vi "Last_L1_FolderName.vi"(11 "folder names":string[](array[string])) -> (3 "File_Name":string[](array[string]))   [LabVIEW 2023]
panel:
  out "Times":i64[](array[numeric])
  out "Name-SN":string[](array[string])
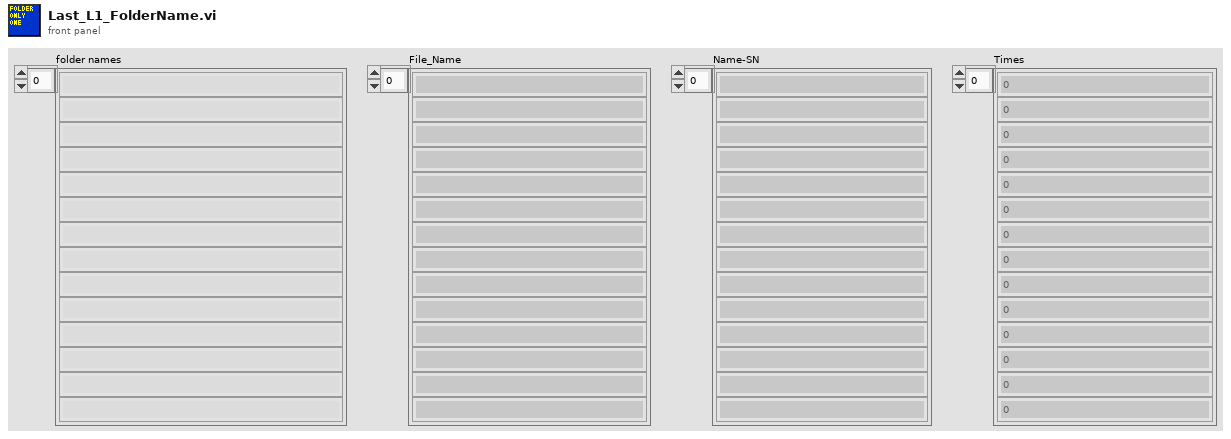
[diagram p1: front panel]
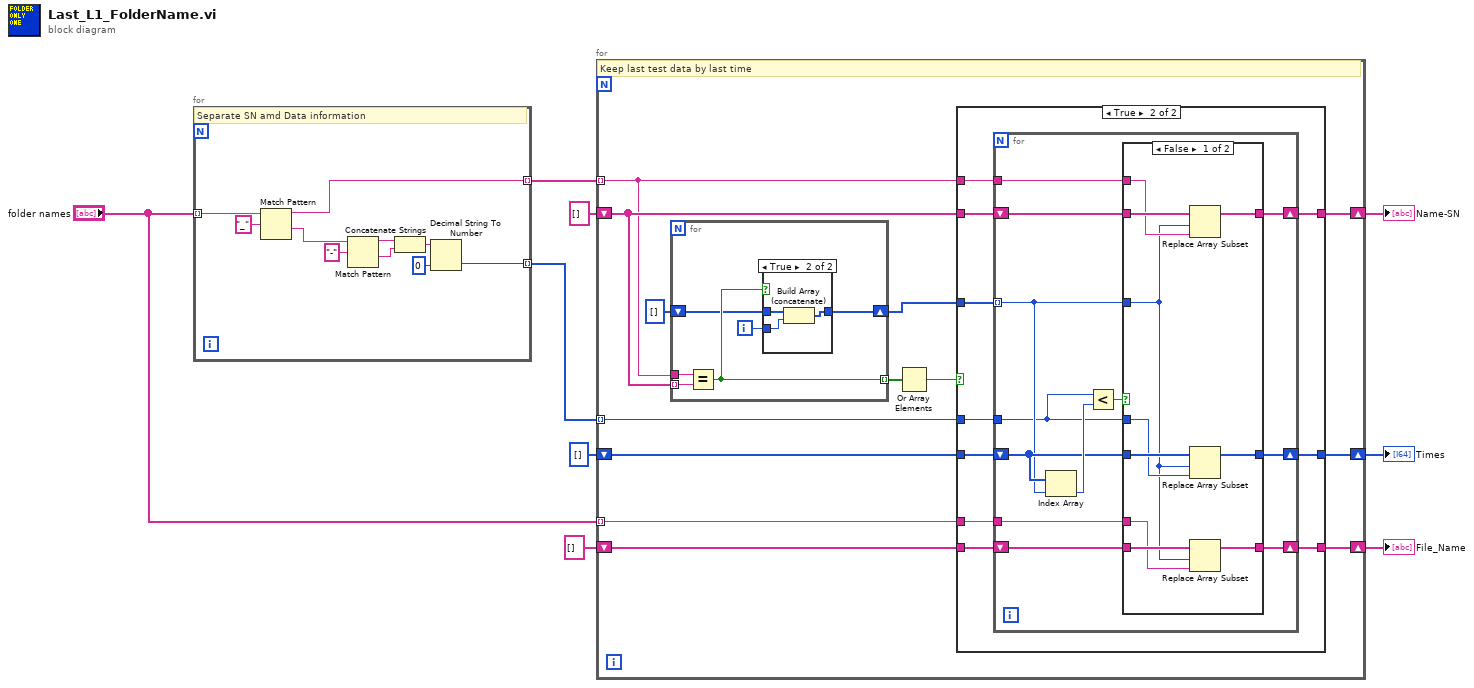
[diagram p0: block diagram]
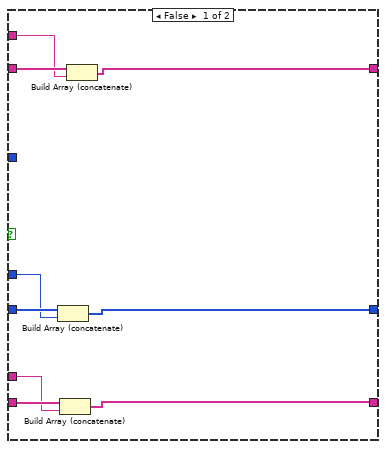
[diagram p2: hidden frame]
diagram:
  n1 = for {
    tunnel: "folder names" -> [w19] mode=indexing
    tunnel: [w12] -> w5 mode=indexing
    tunnel: [w11] -> w4 mode=indexing
    # "Separate SN amd Data information"
    n2 = Match Pattern(string=w19, regular expression="_") -> (before substring=w12:string, after substring=w10:string)  [unwired: 1 in, 2 out]
    n3 = Match Pattern(string=w10, regular expression="-") -> (before substring=w16:string, after substring=w15:string)  [unwired: 1 in, 2 out]
    n4 = Concatenate Strings(w16, w15) -> (w13:string)
    n5 = Decimal String To Number(string=w13, default (0L)=i64 0 ("default (0 I32)")) -> (number=w11:i64)  [unwired: 1 in, 1 out]
  }
  n6 = for {
    tunnel: w5 -> [w27] mode=indexing
    tunnel: w4 -> [w29] mode=indexing
    shift-right: [w26] -> w7
    shift-left: string[] [] -> [w28]
    shift-right: [w25] -> w6
    shift-left: i64[] [] -> [w30]
    tunnel: "folder names" -> [w22] mode=indexing
    shift-right: [w20] -> w2
    shift-left: string[] [] -> [w21]
    # "Keep last test data by last time"
    n7 = for {
      tunnel: w27 -> [w82]
      tunnel: w28 -> [w81] mode=indexing
      tunnel: [w80] -> w32 mode=indexing
      shift-right: [w77] -> w23
      shift-left: i32[] [] -> [w78]
      i -> [w79]
      n8 = Equal?(x=w82, y=w81) -> (x = y?=w80:bool)
      n9 = case shown="True" w80 {
        tunnel: w79 -> [_ w85]
        tunnel: w78 -> [w83 w86]
        tunnel: [w83 w84] -> w77
        frame False {
        }
        frame True {
          n10 = Build Array (concatenate)(w86, w85) -> (w84:i32[])
        }
      }
    }
    n11 = Or Array Elements(Boolean array=w32) -> (logical OR=w31:bool)
    n12 = case shown="True" w31 {
      tunnel: w30 -> [w38 w50]
      tunnel: w29 -> [w37 w49]
      tunnel: w28 -> [w41 w48]
      tunnel: w27 -> [w40 w45]
      tunnel: [w39 w47] -> w26
      tunnel: [w36 w46] -> w25
      tunnel: w23 -> [_ w51]
      tunnel: w22 -> [w34 w44]
      tunnel: w21 -> [w35 w43]
      tunnel: [w33 w42] -> w20
      frame False {
        n13 = Build Array (concatenate)(w38, w37) -> (w36:i64[])
        n14 = Build Array (concatenate)(w35, w34) -> (w33:string[])
        n15 = Build Array (concatenate)(w41, w40) -> (w39:string[])
      }
      frame True {
        n16 = for {
          tunnel: w51 -> [w57] mode=indexing
          shift-right: [w58] -> w46
          shift-left: w50 -> [w59]
          tunnel: w49 -> [w55]
          shift-right: [w60] -> w47
          shift-left: w48 -> [w61]
          tunnel: w45 -> [w56]
          tunnel: w44 -> [w54]
          shift-right: [w52] -> w42
          shift-left: w43 -> [w53]
          n17 = Index Array(array=w59, index=w57) -> (element=w63:i64)
          n18 = Less?(x=w55, y=w63) -> (x < y?=w62:bool)
          n19 = case shown="False" w62 {
            tunnel: w61 -> [w73 w76]
            tunnel: [w69 w76] -> w60
            tunnel: w59 -> [w72 w75]
            tunnel: [w68 w75] -> w58
            tunnel: w57 -> [w65 _]
            tunnel: w56 -> [w71 _]
            tunnel: w55 -> [w70 _]
            tunnel: w54 -> [w66 _]
            tunnel: w53 -> [w67 w74]
            tunnel: [w64 w74] -> w52
            frame False {
              n20 = Replace Array Subset(array=w73, new element=w71, index=w65) -> (w69:string[])
              n21 = Replace Array Subset(array=w72, new element=w70, index=w65) -> (w68:i64[])
              n22 = Replace Array Subset(array=w67, new element=w66, index=w65) -> (w64:string[])
            }
            frame True {
            }
          }
        }
      }
    }
  }
  "Name-SN" <- w7
  "Times" <- w6
  "File_Name" <- w2
